vi "33 GPS Time to Labview Time (2017).vi"(1 "GPS Date":string, 2 "GPS Time":string) -> (0 "Labview Time Stamp":timestamp)   [LabVIEW 2017]
panel:
  in  "Century":dbl
  # "HR:MM:SS.MSS"
  # "MM/DD/YY"
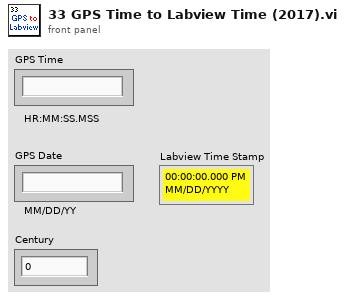
[diagram p1: front panel]
types:
  T1 = cluster{"second":i32, "minute":i32, "hour":i32, "day of month":i32, "month":i32, "year":i32, "day of week":i32, "day of year":i32, "is DST":i32}
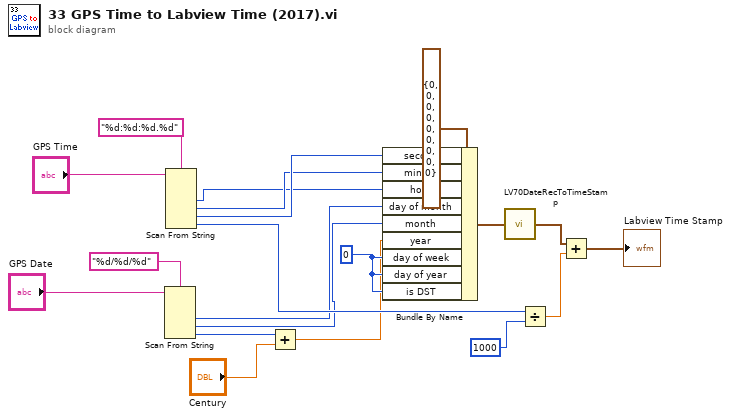
[diagram p0: block diagram]
diagram:
  w9 = 0
  n1 = Scan From String "Scan From String"(format string="%d/%d/%d", input string="GPS Date") -> (output 1=w7:i32, output 2=w6:i32, output 3=w5:i32)  [unwired: 5 in, 3 out]
  n2 = Scan From String "Scan From String"(format string="%d:%d:%d.%d", input string="GPS Time") -> (output 1=w10:i32, output 2=w11:i32, output 3=w12:i32, output 4=w14:i32)  [unwired: 6 in, 3 out]
  n3 = Add(x=w5, y="Century") -> (x+y=w4:dbl)
  n4 = Bundle By Name(cluster=T1 {"second"=0, "minute"=0, "hour"=0, "day of month"=0, "month"=0, "year"=0, "day of week"=0, "day of year"=0, "is DST"=0} ("date time rec"), "second"=w12, "minute"=w11, "hour"=w10, "day of month"=w7, "month"=w6, "year"=w4, "day of week"=w9, "day of year"=w9, "is DST"=w9) -> (w19:T1)
  n5 = call <vilib>:"LV70DateRecToTimeStamp.vi"("date time rec"=w19) -> ("Time Stamp"=w17:timestamp)
  n6 = Divide(x=w14, y=1000) -> (x/y=w15:dbl)
  n7 = Add(x=w17, y=w15) -> (x+y=→"Labview Time Stamp":timestamp)
